vi "Measure Fringe Displacement.vi"(0 "Photodiode Output":dbl, 7 "Fringe Counter Settings":T1={"Wavelength"=6e-07, "Divisions"=2.0, "Scaling Amplitude"=1.2, "Scaling Offset"=0.0} {"Scaling Offset" format="%0.2f"; "Scaling Amplitude" format="%0.2f"}, 9 "Reset":bool) -> (4 "Displacement":dbl=6e-06, 6 "Input Signals":dbl[][](graph), 8 "Stepped Signal":dbl(graph), 10 "Output Signal":dbl[](graph), 15 "Initial Step Position":dbl)   [LabVIEW 2013]
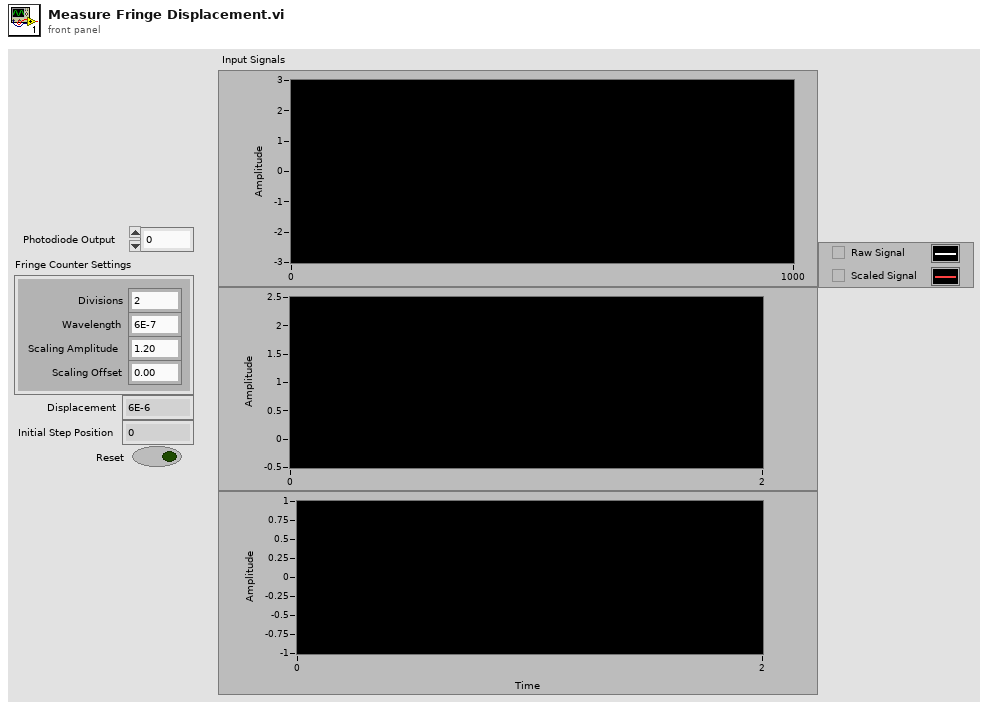
[diagram p1: front panel]
types:
  T1 = cluster{"Wavelength":dbl, "Divisions":dbl, "Scaling Amplitude":dbl, "Scaling Offset":dbl}
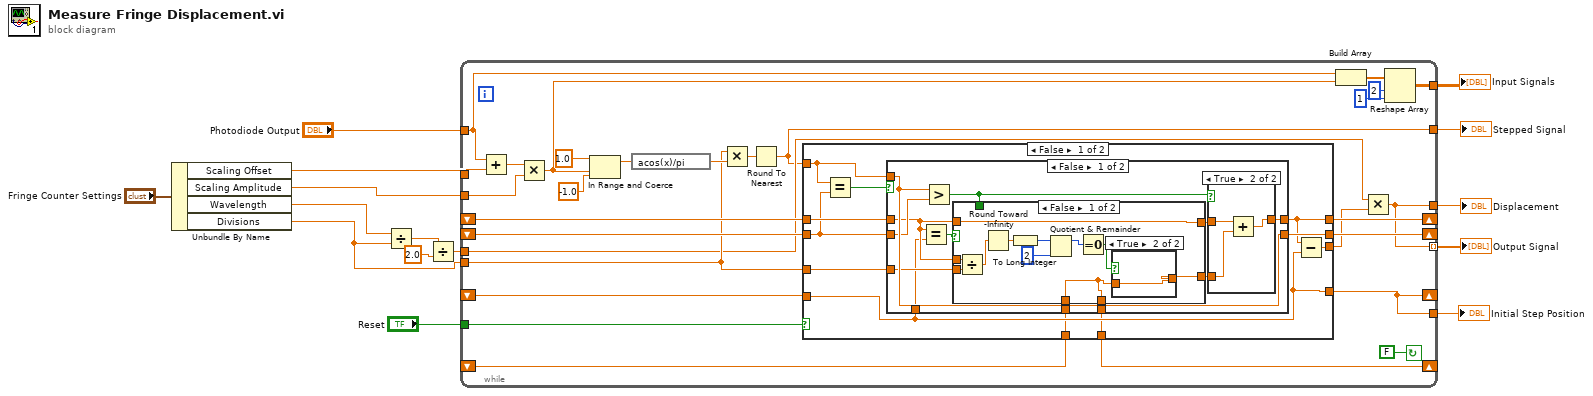
[diagram p0: block diagram]
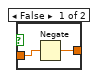
[diagram p2: hidden frame]
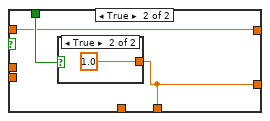
[diagram p3: hidden frame]
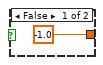
[diagram p4: hidden frame]
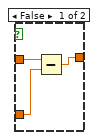
[diagram p5: hidden frame]
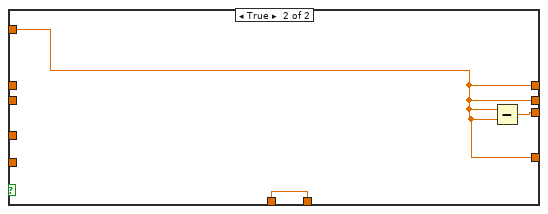
[diagram p7: hidden frame]
diagram:
  n1 = Unbundle By Name("Fringe Counter Settings") -> ("Scaling Offset"=w4:dbl, "Scaling Amplitude"=w3:dbl, "Wavelength"=w2:dbl, "Divisions"=w1:dbl)
  n2 = Divide(x=w2, y=w1) -> (x/y=w6:dbl)
  n3 = Divide(x=w6, y=2.0) -> (x/y=w8:dbl)
  n4 = while {
    tunnel: [w34] -> w10 mode=indexing
    shift-right: [w35] -> _
    shift-left: _ -> [w43]
    shift-right: [w37] -> _
    shift-left: _ -> [w44]
    tunnel: w1 -> [w36]
    tunnel: [w34] -> w9
    tunnel: w8 -> [w33]
    tunnel: w4 -> [w30]
    tunnel: w3 -> [w29]
    tunnel: [w27] -> w11
    tunnel: [w22] -> w12
    tunnel: "Photodiode Output" -> [w21]
    shift-right: [w19] -> _
    shift-left: _ -> [w20]
    tunnel: [w19] -> w14
    shift-right: [w18] -> _
    shift-left: _ -> [w17]
    tunnel: "Reset" -> [w16]
    stop <- FALSE continue-if-true
    n5 = Add(x=w21, y=w30) -> (x+y=w31:dbl)
    n6 = Multiply(x=w31, y=w29) -> (x*y=w26:dbl)
    n7 = In Range and Coerce(upper limit=1.0, x=w26, lower limit=-1.0) -> (coerced(x)=w40:dbl)  [unwired: 1 out]
    n8 = expression code="acos(x)/pi"(w40) -> (w41:dbl)
    n9 = Multiply(x=w36, y=w41) -> (x*y=w42:dbl)
    n10 = Round To Nearest(number=w42) -> (nearest integer value=w27:dbl)
    n11 = case shown="False" w16 {
      tunnel: w44 -> [w53 _]
      tunnel: w43 -> [w54 _]
      tunnel: w36 -> [w50 _]
      tunnel: w27 -> [w51 w97]
      tunnel: [w52 w97] -> w37
      tunnel: [w48 w97] -> w35
      tunnel: [w49 w98] -> w32
      tunnel: w20 -> [w47 _]
      tunnel: [w47 w97] -> w19
      tunnel: [w46 w96] -> w18
      tunnel: w17 -> [w45 w96]
      frame False {
        n12 = Equal?(x=w51, y=w53) -> (x = y?=w55:bool)
        n13 = case shown="False" w55 {
          tunnel: [w66 w95] -> w48
          tunnel: w54 -> [w60 w95]
          tunnel: w53 -> [w61 w94]
          tunnel: [w65 w94] -> w52
          tunnel: w51 -> [w65 _]
          tunnel: w50 -> [w64 _]
          tunnel: w47 -> [w58 _]
          tunnel: [w57 w93] -> w46
          tunnel: w45 -> [w56 w93]
          frame False {
            n14 = Equal?(x=w60, y=w58) -> (x = y?=w62:bool)
            n15 = Greater?(x=w65, y=w61) -> (0:w59:bool)
            n16 = case shown="False" w62 {
              tunnel: [w78 w82] -> w67
              tunnel: w60 -> [w77 _]
              tunnel: w64 -> [w76 _]
              tunnel: [w69 w83] -> w63
              tunnel: w60 -> [w69 w83]
              tunnel: w59 -> [_ w84]
              tunnel: [w68 w82] -> w57
              tunnel: w56 -> [w68 _]
              frame False {
                n17 = Divide(x=w77, y=w76) -> (x/y=w75:dbl)
                n18 = Round Toward -Infinity(1:w75) -> (0:w74:dbl)
                n19 = To Long Integer(number=w74) -> (32bit integer=w73:i32)
                n20 = Quotient & Remainder(x=w73, y=2) -> (x-y*floor(x/y)=w70:i32)  [unwired: 1 out]
                n21 = Equal To 0?(x=w70) -> (x = 0?=w71:bool)
                n22 = case shown="True" w71 {
                  tunnel: [w80 w81] -> w78
                  tunnel: w68 -> [w79 w81]
                  frame False {
                    n23 = Negate(x=w79) -> (-x=w80:dbl)
                  }
                  frame True {
                  }
                }
              }
              frame True {
                n24 = case shown="True" w84 {
                  tunnel: [-1.0 1.0] -> w82
                  frame False {
                  }
                  frame True {
                  }
                }
              }
            }
            n25 = case shown="True" w59 {
              tunnel: w67 -> [w88 w92]
              tunnel: w63 -> [w87 w91]
              tunnel: [w89 w90] -> w66
              frame False {
                n26 = Subtract(x=w87, y=w88) -> (x-y=w89:dbl)
              }
              frame True {
                n27 = Add(x=w91, y=w92) -> (x+y=w90:dbl)
              }
            }
          }
          frame True {
          }
        }
        n28 = Subtract(x=w48, y=w47) -> (x-y=w49:dbl)
      }
      frame True {
        n29 = Subtract(x=w97, y=w97) -> (x-y=w98:dbl)
      }
    }
    n30 = Build Array(w21, w26) -> (w25:dbl[])
    n31 = Multiply(x=w33, y=w32) -> (x*y=w34:dbl)
    n32 = Reshape Array(w25, 2 ("dimension size"), 1 ("dimension size")) -> (w22:dbl[][])
  }
  "Output Signal" <- w10
  "Displacement" <- w9
  "Stepped Signal" <- w11
  "Input Signals" <- w12
  "Initial Step Position" <- w14
